vi "Align stuckbead signal.vi"(3 "avg range for QPD center (nm)":dbl=600.0, 4 "stuckbstuck QPD (V)":dbl[](array[numeric]), 5 "Stage (um)":dbl[](array[numeric]), 6 "Read data?":bool) -> (0 "Aligned QPD (V)":dbl[](array[numeric]), 2 "Bead radius (nm)":dbl[](array[numeric]))   [LabVIEW 2014]
panel:
  out "Guess-stage-center (um)":dbl
  out "Guess-QPD-center (V)":dbl
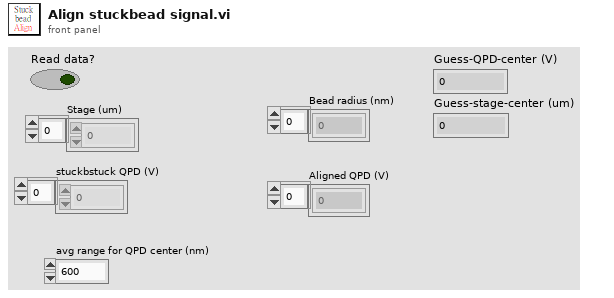
[diagram p1: front panel]
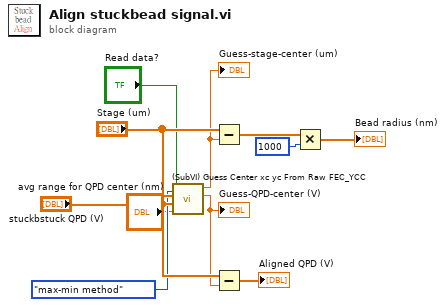
[diagram p0: block diagram]
diagram:
  n1 = call "(SubVI) Guess Center xc yc From Raw FEC_YCC.vi"("Enum"=enum16{"parity method", "max-min method"}."max-min method", "avg range for QPD center (nm)"="avg range for QPD center (nm)", "QPD array (V)"="stuckbstuck QPD (V)", "Stage array(um)"="Stage (um)", "Read data?"="Read data?") -> ("Guess-QPD-center (V)"=w3:dbl, "Guess-stage-center(um)"=w4:dbl)  [unwired: 1 in, 2 out]
  "Guess-QPD-center (V)" <- w3
  "Guess-stage-center (um)" <- w4
  n2 = Subtract(x="Stage (um)", y=w4) -> (x-y=w11:dbl[])
  n3 = Subtract(x="stuckbstuck QPD (V)", y=w3) -> (x-y=→"Aligned QPD (V)":dbl[])
  n4 = Multiply(x=w11, y=1000 ("index (col)")) -> (x*y=→"Bead radius (nm)":dbl[])
